vi "Add_Part_of_Track(101)-1.vi"(5 "[IN] Minimal Sub\ntrack Length":i32, 6 "[IN] Index in subtrack":i32, 7 "[IN] # of subtrack conta\nining problem point":i32, 8 "error IN":errorcluster, 9 "[IN] Subtrack":T1, 10 "[IN] Index of problem\npoint inside subtrack":i32, 11 "[IN] Still connected\ntracks in group":T2) -> (0 "error OUT":errorcluster, 1 "[OUT] Subtrack":T1, 3 "[OUT] Last point in subtrack":i32)   [LabVIEW 2013]
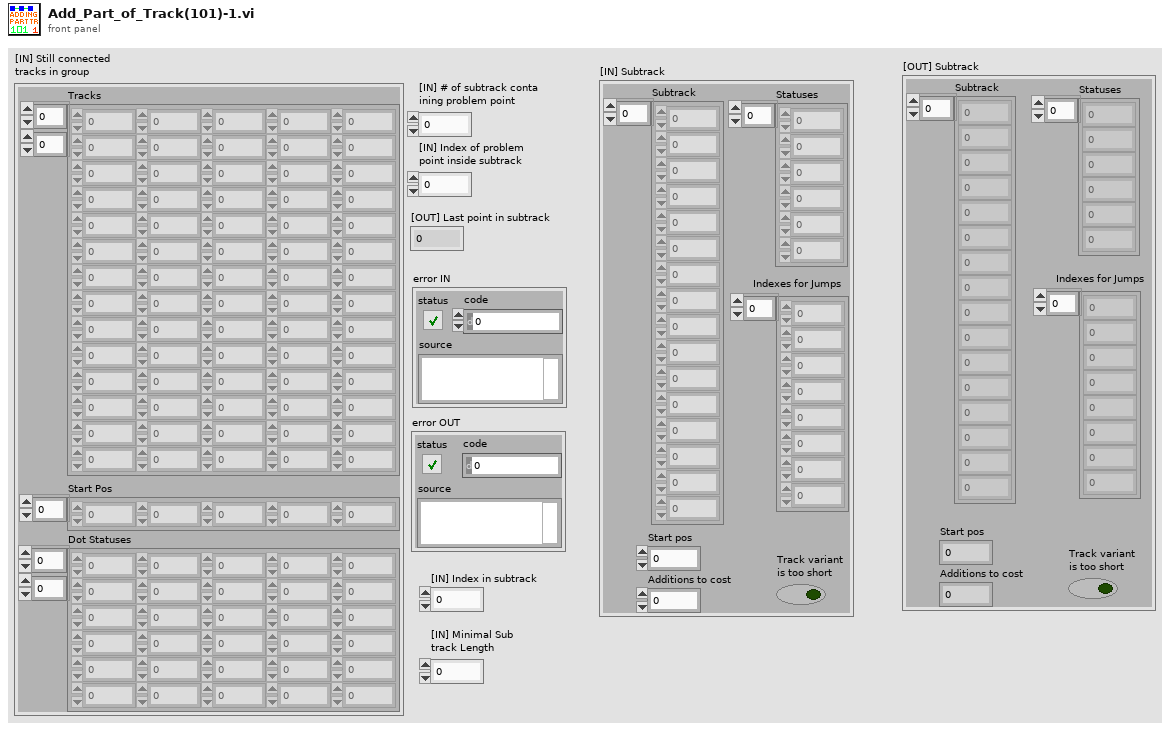
[diagram p1: front panel]
types:
  T1 = cluster{"Subtrack":dbl[], "Statuses":i16[], "Start pos":i32, "Additions to cost":i32, "Track variant \nis too short":bool, "Indexes for Jumps":i32[]}
  T2 = cluster{"Tracks":dbl[][], "Start Pos":i32[], "Dot Statuses":i16[][]}
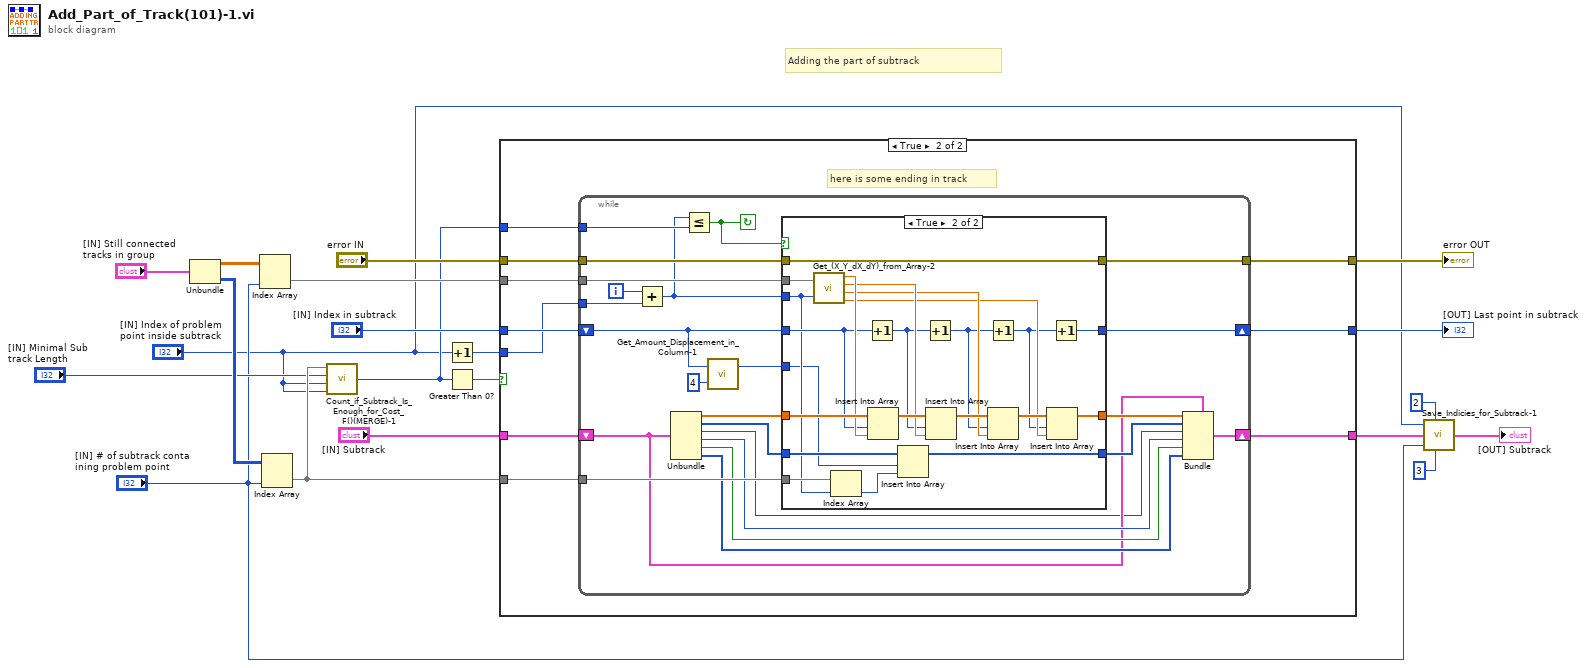
[diagram p0: block diagram]
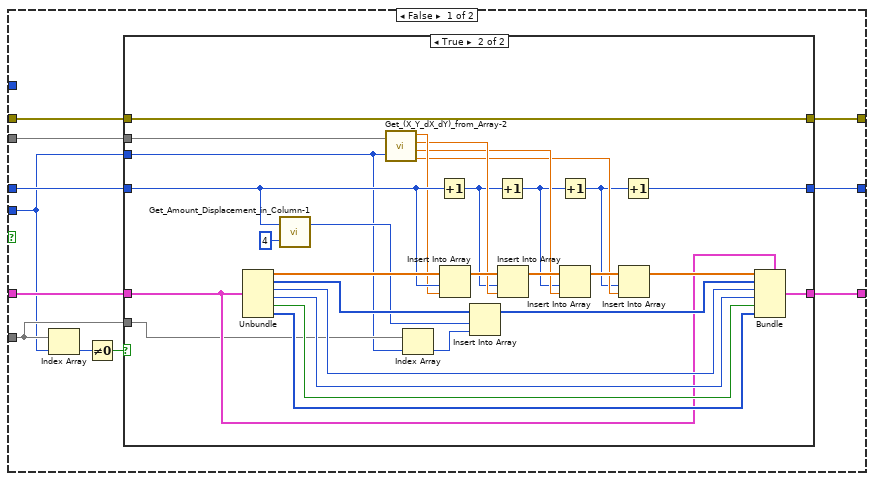
[diagram p2: hidden frame]
diagram:
  # "Adding the part of subtrack"
  n1 = Unbundle("[IN] Still connected\ntracks in group") -> ("Tracks"=w18:dbl[][], "Dot Statuses"=w16:i16[][])  [unwired: 1 out]
  n2 = Index Array(array=w18, index (col)="[IN] # of subtrack conta\nining problem point") -> (element=w17:dbl[])  [unwired: 1 in]
  n3 = Index Array(array=w16, index (col)="[IN] # of subtrack conta\nining problem point") -> (element=w9:i16[])  [unwired: 1 in]
  n4 = call "Count_if_Subtrack_Is_Enough_for_Cost_F()(MERGE)-1.vi"("[IN] Index of Earliest \nProblem Point Inside\nFisrt Part of Track"="[IN] Index of problem\npoint inside subtrack", "[IN] Index of Problem \nPoint Inside Second Track"="[IN] Index of problem\npoint inside subtrack", "[IN] Minimal Subtrack Length \n(Points without problems) for\nMaking Desicion"="[IN] Minimal Sub\ntrack Length", "[IN] Track Statuses in second\npart for track making"=w9) -> ("[OUT] Index of Last \nPoint in Second Track"=w7:i32)  [unwired: 1 in, 1 out]
  n5 = Increment(x="[IN] Index of problem\npoint inside subtrack") -> (x+1=w10:i32)
  n6 = Greater Than 0?(x=w7) -> (x > 0?=w11:bool)
  n7 = case shown="True" w11 {
    tunnel: "error IN" -> [w24 w73]
    tunnel: w17 -> [w23 w72]
    tunnel: [w26 w71] -> w15
    tunnel: [w21 w70] -> w14
    tunnel: "[IN] Subtrack" -> [w29 w69]
    tunnel: "[IN] Index in subtrack" -> [w28 w68]
    tunnel: w9 -> [w25 w67]
    tunnel: w7 -> [_ w66]
    tunnel: w10 -> [w22 w65]
    tunnel: [w27 w64] -> w6
    frame False {
      n8 = Index Array(array=w25, index=w22) -> (element=w31:i16)
      n9 = Not Equal To 0?(x=w31) -> (x != 0?=w30:bool)
      n10 = case shown="True" w30 {
        tunnel: w29 -> [w32 w53]
        tunnel: w28 -> [w33 w52]
        tunnel: [w32 w51] -> w27
        tunnel: [w33 w50] -> w26
        tunnel: w25 -> [_ w49]
        tunnel: w24 -> [w34 w35]
        tunnel: w23 -> [_ w48]
        tunnel: w22 -> [_ w47]
        tunnel: [w34 w35] -> w21
        frame False {
        }
        frame True {
          n11 = Unbundle(w53) -> ("Subtrack"=w63:dbl[], "Statuses"=w62:i16[], "Start pos"=w54:i32, "Additions to cost"=w59:i32, "Track variant \nis too short"=w58:bool, "Indexes for Jumps"=w57:i32[])
          n12 = call "Get_Amount_Displacement_in_Column-1.vi"("multiplier"=4, "# Rows"=w52) -> ("Displ amount"=w55:i32)  [unwired: 1 out]
          n13 = call "Get_(X_Y_dX_dY)_from_Array-2.vi"("(X,Y,dX,dY)"=w48, "Index of Displacement"=w47) -> ("X"=w46:dbl, "Y"=w44:dbl, "dX"=w41:dbl, "dY"=w38:dbl)
          n14 = Index Array(array=w49, index=w47) -> (element=w37:i16)
          n15 = Increment(x=w52) -> (x+1=w42:i32)
          n16 = Insert Into Array(array=w63, index=w52, new element=w46) -> (w45:dbl[])
          n17 = Insert Into Array(array=w62, index=w55, new element=w37) -> (w60:i16[])
          n18 = Increment(x=w42) -> (x+1=w40:i32)
          n19 = Insert Into Array(array=w45, index=w42, new element=w44) -> (w43:dbl[])
          n20 = Increment(x=w40) -> (x+1=w36:i32)
          n21 = Insert Into Array(array=w43, index=w40, new element=w41) -> (w39:dbl[])
          n22 = Insert Into Array(array=w39, index=w36, new element=w38) -> (w61:dbl[])
          n23 = Increment(x=w36) -> (x+1=w50:i32)
          n24 = Bundle(cluster=w53, "Subtrack"=w61, "Statuses"=w60, "Start pos"=w54, "Additions to cost"=w59, "Track variant \nis too short"=w58, "Indexes for Jumps"=w57) -> (w51:T1)
        }
      }
    }
    frame True {
      # "here is some ending in track"
      n25 = while {
        tunnel: w72 -> [w96]
        tunnel: w67 -> [w92]
        shift-right: [w89] -> w64
        shift-left: w69 -> [w83]
        tunnel: w73 -> [w85]
        tunnel: [w84] -> w70
        shift-right: [w82] -> w71
        shift-left: w68 -> [w80]
        tunnel: w66 -> [w77]
        tunnel: w65 -> [w74]
        i -> [w76]
        stop <- w94 continue-if-true
        n26 = Add(x=w76, y=w74) -> (x+y=w75:i32)
        n27 = Unbundle(w83) -> ("Subtrack"=w95:dbl[], "Statuses"=w93:i16[], "Start pos"=w78:i32, "Additions to cost"=w88:i32, "Track variant \nis too short"=w87:bool, "Indexes for Jumps"=w86:i32[])
        n28 = Less Or Equal?(x=w75, y=w77) -> (x <= y?=w94:bool)
        n29 = call "Get_Amount_Displacement_in_Column-1.vi"("multiplier"=4, "# Rows"=w80) -> ("Displ amount"=w79:i32)  [unwired: 1 out]
        n30 = case shown="True" w94 {
          tunnel: w96 -> [_ w122]
          tunnel: w95 -> [w99 w121]
          tunnel: w80 -> [w97 w119]
          tunnel: w75 -> [_ w108]
          tunnel: w93 -> [w100 w110]
          tunnel: w92 -> [_ w109]
          tunnel: [w99 w106] -> w91
          tunnel: [w100 w105] -> w90
          tunnel: w85 -> [w98 w104]
          tunnel: [w98 w104] -> w84
          tunnel: [w97 w101] -> w82
          tunnel: w79 -> [_ w103]
          frame False {
          }
          frame True {
            n31 = call "Get_(X_Y_dX_dY)_from_Array-2.vi"("(X,Y,dX,dY)"=w122, "Index of Displacement"=w108) -> ("X"=w120:dbl, "Y"=w117:dbl, "dX"=w114:dbl, "dY"=w111:dbl)
            n32 = Index Array(array=w109, index=w108) -> (element=w107:i16)
            n33 = Increment(x=w119) -> (x+1=w115:i32)
            n34 = Insert Into Array(array=w121, index=w119, new element=w120) -> (w118:dbl[])
            n35 = Insert Into Array(array=w110, index=w103, new element=w107) -> (w105:i16[])
            n36 = Increment(x=w115) -> (x+1=w113:i32)
            n37 = Insert Into Array(array=w118, index=w115, new element=w117) -> (w116:dbl[])
            n38 = Increment(x=w113) -> (x+1=w102:i32)
            n39 = Insert Into Array(array=w116, index=w113, new element=w114) -> (w112:dbl[])
            n40 = Insert Into Array(array=w112, index=w102, new element=w111) -> (w106:dbl[])
            n41 = Increment(x=w102) -> (x+1=w101:i32)
          }
        }
        n42 = Bundle(cluster=w83, "Subtrack"=w91, "Statuses"=w90, "Start pos"=w78, "Additions to cost"=w88, "Track variant \nis too short"=w87, "Indexes for Jumps"=w86) -> (w89:T1)
      }
    }
  }
  "[OUT] Last point in subtrack" <- w15
  "error OUT" <- w14
  n43 = call "Save_Indicies_for_Subtrack-1.vi"("[IN] Index of Origin/Problem \nPoint inside Original Track (X1)"="[IN] Index of problem\npoint inside subtrack", "[IN] i for X1"=2, "[IN] Subtrack"=w6, "[IN] Index of Track Conta-\nining Origin/Problem (X2)"="[IN] # of subtrack conta\nining problem point", "[IN] i for X2"=3 ("[IN] i for X1")) -> ("[OUT] Subtrack"=→"[OUT] Subtrack":T1)
